vi "Set CPTR Period.vi"(0 "Register Buses":refnum<class "ni579x Register Bus v1 Host.lvclass">[](array[class]), 5 "sync.cptr.period":u16[](array[numeric]), 11 "error in":errorcluster) -> (4 "Register Buses (out)":refnum<class "ni579x Register Bus v1 Host.lvclass">[](array[class]), 15 "error out":errorcluster)   [LabVIEW 2012, in "ni579x Synchronization v1 Host.lvlib"]
uses:
  <instrlib>/ni579x/Synchronization/v1/Host/ni579x Synchronization v1 Host.lvlib
  <instrlib>/ni579x/Register Bus/v1/Host/ni579x Register Bus v1 Host.lvclass
  <instrlib>/ni579x/Synchronization/v1/Shared/ni579x Synchronization Register Addresses.ctl
  <instrlib>/ni579x/Register Bus/v1/Host/Public/Register Write.ctl
  <instrlib>/ni579x/Config/v1/Shared/Types/ni579x Register Bus Subsystem ID.ctl
  <vilib>/Utility/error.llb/Error Cluster From Error Code.vi
  <vilib>/ErrorRing/Error Ring.xnode
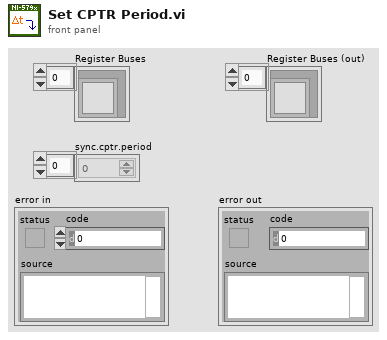
[diagram p1: front panel]
types:
  T1 = typedef "ni579x Register Bus v1 Host.lvclass/Register Write.ctl" = cluster{"subsystem":u8, "address":u16, "data":u32}
  T2 = typedef "ni579x Synchronization Register Addresses.ctl" = enum16{"Signature", "Current Version", "Oldest Compatible Version", "Scratch Register", "sync.master", "sync.meas.enable", "sync.meas.ready", "sync.meas.arm", "sync.meas.valid", "sync.meas.value", "sync.cptr.adjust", "sync.cptr.period", "sync.meas.oversample factor"}
  T3 = typedef "ni579x Register Bus Subsystem ID.ctl" = u8
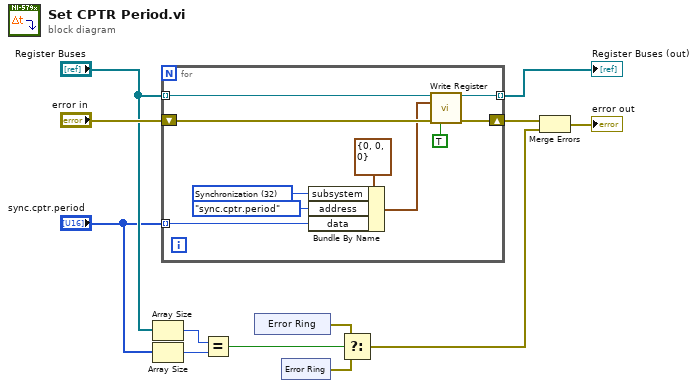
[diagram p0: block diagram]
diagram:
  n1 = Array Size(array="Register Buses") -> (size(s)=w9:i32)
  n2 = Array Size(array="sync.cptr.period") -> (size(s)=w8:i32)
  n3 = for {
    tunnel: "Register Buses" -> [w22] mode=indexing
    tunnel: [w19] -> w1 mode=indexing
    shift-right: [w18] -> w4
    shift-left: "error in" -> [w21]
    tunnel: "sync.cptr.period" -> [w13] mode=indexing
    w16 = T3 32 items=["FAM Register Operation"=0, "User Command"=16, "Synchronization"=32] ("Subsystem ID")
    n4 = Bundle By Name(cluster=T1 {"subsystem"=0, "address"=0, "data"=0} ("register write"), "subsystem"=w16, "address"=ni579x_Synchronization_Register_Addresses."sync.cptr.period" ("Synchronization Registers"), "data"=w13) -> (w14:T1)
    n5 = call <instrlib>:"Write Register.vi"("session in"=w22, "register write"=w14, "error in"=w21, "wait until committed"=TRUE) -> ("session out"=w19:refnum<class "ni579x Register Bus v1 Host.lvclass">, "error out"=w18:errorcluster)  [unwired: 10 in]
  }
  "Register Buses (out)" <- w1
  n6 = Equal?(x=w9, y=w8) -> (x = y?=w7:bool)
  n7 = xnode "Error Ring"() -> ("error out"=w6:errorcluster)
  n8 = xnode "Error Ring"() -> ("error out"=w5:errorcluster)
  n9 = Select(t=w6, s=w7, f=w5) -> (s? t:f=w2:errorcluster)
  n10 = Merge Errors(w4, w2) -> (→"error out":errorcluster)
